vi "SetFillLevel.vi"(0 "object in":refnum<class "CetoniPump.lvclass">, 1 "index":i32, 2 "Flow":dbl, 3 "Level(ml)":dbl, 5 "error in (no error)":errorcluster) -> (14 "object out":refnum<class "CetoniPump.lvclass">, 16 "Values Not Permitted":bool, 17 "Coerced Level":dbl, 18 "Coerced Flow":dbl, 19 "error out":errorcluster)   [LabVIEW 2021, in "CetoniPump.lvclass"]
uses:
  CetoniPump.lvclass
  CetoniPump.lvclass/CetoniPump.ctl
  Users/olaja/AppData/Local/CETONI_SDK/lib/labview/labbCAN_Pump_API/labbCAN_Pump_API.lvlib
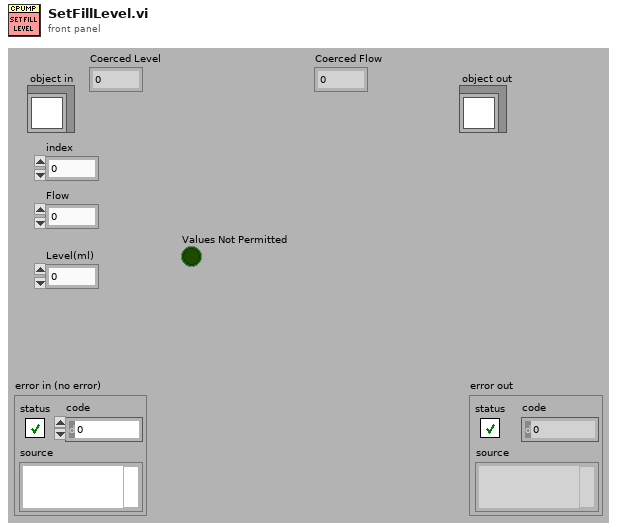
[diagram p1: front panel]
types:
  T1 = cluster{"Pump Handle":i64, "Pump Name":string, "Maximum Volume":dbl, "Maximum Flow Rate":dbl, "Flow Rate":dbl, "Target Level":dbl}[]
  T2 = cluster{"Pump Handle":i64, "Pump Name":string, "Maximum Volume":dbl, "Maximum Flow Rate":dbl, "Flow Rate":dbl, "Target Level":dbl}
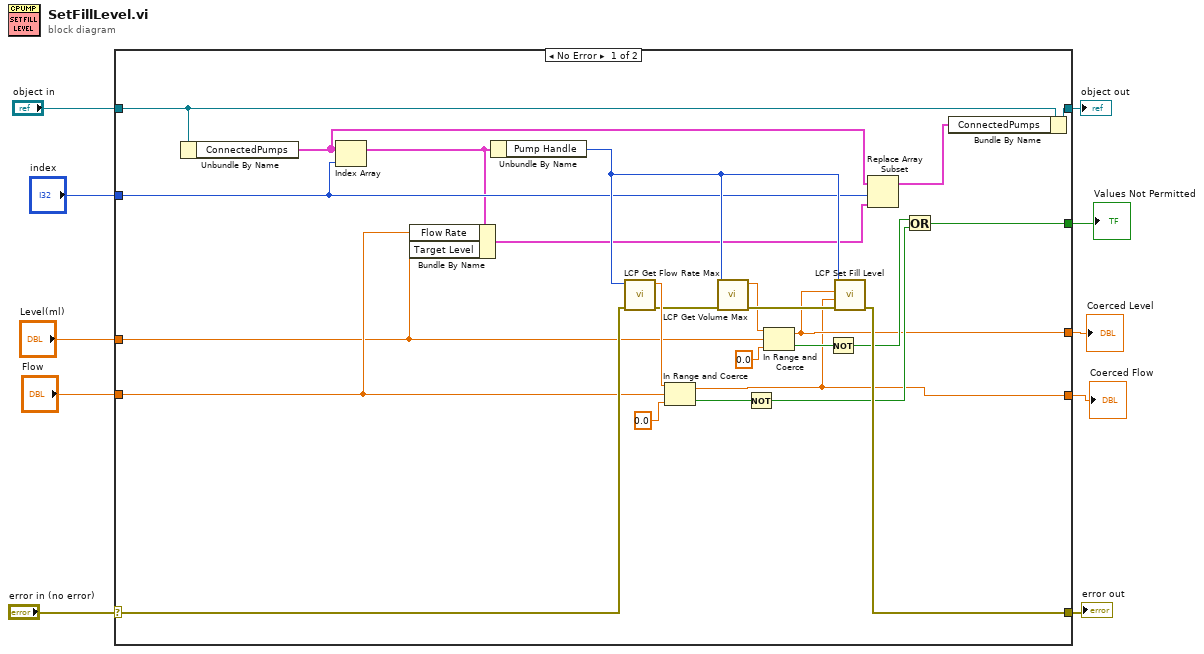
[diagram p0: block diagram]
diagram:
  n1 = case shown="No Error" "error in (no error)" {
    selector: "error in (no error)" -> [w31 w37]
    tunnel: [w34 w37] -> w9
    tunnel: [w14 w36] -> w7
    tunnel: "object in" -> [w35 w36]
    tunnel: "Level(ml)" -> [w17 _]
    tunnel: "Flow" -> [w18 _]
    tunnel: "index" -> [w20 _]
    tunnel: [w21 _] -> w3
    tunnel: [w12 _] -> w2
    tunnel: [w11 _] -> w1
    frame No Error {
      n2 = Unbundle By Name(w35) -> ("ConnectedPumps"=w16:T1)
      n3 = Index Array(array=w16, index=w20) -> (element=w19:T2)
      n4 = Bundle By Name(cluster=w19, "Flow Rate"=w18, "Target Level"=w17) -> (w15:T2)
      n5 = Unbundle By Name(w19) -> ("Pump Handle"=w33:i64)
      n6 = call "LCP Get Flow Rate Max.vi"("error in (no error)"=w31, "Pump Handle"=w33) -> ("error out"=w30:errorcluster, "Maximum Flow Rate"=w32:dbl)  [unwired: 8 in]
      n7 = In Range and Coerce(upper limit=w32, x=w18, lower limit=0.0) -> (coerced(x)=w11:dbl, In Range?=w25:bool)
      n8 = call "LCP Get Volume Max.vi"("error in (no error)"=w30, "Pump Handle"=w33) -> ("error out"=w29:errorcluster, "Maximum Volume"=w28:dbl)  [unwired: 8 in]
      n9 = Not(x=w25) -> (.not. x?=w22:bool)
      n10 = In Range and Coerce(upper limit=w28, x=w17, lower limit=0.0) -> (coerced(x)=w12:dbl, In Range?=w24:bool)
      n11 = Not(x=w24) -> (.not. x?=w23:bool)
      n12 = call "LCP Set Fill Level.vi"("error in (no error)"=w29, "Flow"=w11, "Level"=w12, "Pump Handle"=w33) -> ("error out"=w34:errorcluster)  [unwired: 7 in]
      n13 = Replace Array Subset(array=w16, new element=w15, index=w20) -> (w13:T1)
      n14 = Or(x=w23, y=w22) -> (x .or. y?=w21:bool)
      n15 = Bundle By Name(cluster=w35, "ConnectedPumps"=w13) -> (w14:refnum<class "CetoniPump.lvclass">)
    }
    frame Error {
    }
  }
  "error out" <- w9
  "object out" <- w7
  "Values Not Permitted" <- w3
  "Coerced Level" <- w2
  "Coerced Flow" <- w1
